vi "Mcp2210 Set Gpio Pin Val.vi"(8 "error in (no error)":errorcluster, 10 "GPIO Output":bool[](array[boolean]), 11 "handle":i32) -> (0 "error out":errorcluster, 2 "GPIO Output out":bool[](array[boolean]), 3 "handle out":i32)   [LabVIEW 2015, in "mcp2210.lvlib"]
doc: "Set the GPIO current values. Also returns back the current values.\nThe values are valid only for the pins previously configured as GPIOs.\nParameters:\nInputs:\n- void *handle - The pointer to the device handle. Cannot be NULL.\n- unsigned int gpioSetVal - GPIO pin new values.\nOutputs:\n- unsigned int *pgpioPinVal - GPIO pin values reported back, if successful call.\nIn case of error the value is not changed.\nCannot be NULL pointer.\nReturns:\n- 0 for success: E_SUCCESS\n- negative error code: E_ERR_NULL, E_ERR_INVALID_HANDLE_VALUE\nE_ERR_UNKOWN_ERROR, E_ERR_INVALID_PARAMETER\nE_ERR_HID_TIMEOUT, E_ERR_HID_RW_FILEIO\nE_ERR_CMD_ECHO, E_ERR_CMD_FAILED\n\nMCP2210_DLL_UM_API int __stdcall Mcp2210_SetGpioPinVal(void *handle, unsigned int gpioSetVal, unsigned int *pgpioPinVal);"
uses:
  <userlib>/mcp2210/mcp2210.lvlib
  <userlib>/mcp2210/mcp2210_dll_um_x86.dll
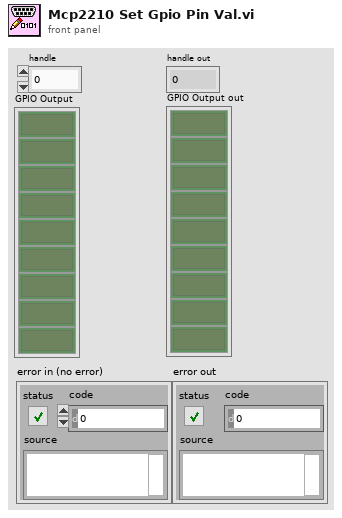
[diagram p1: front panel]
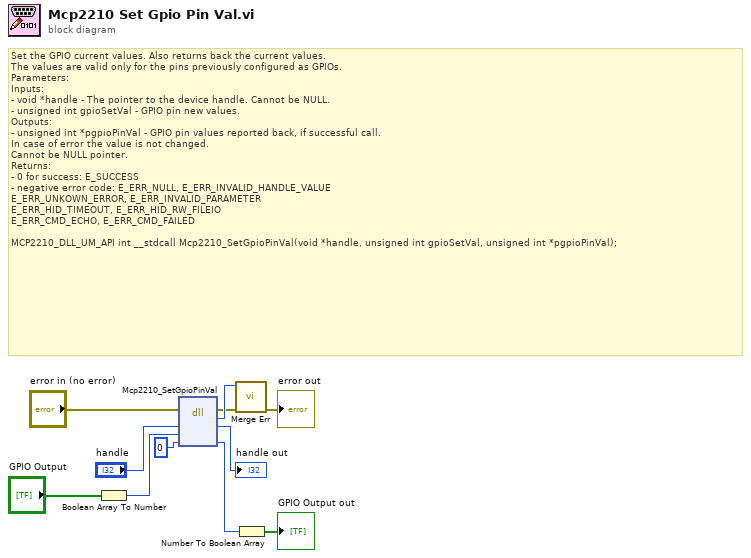
[diagram p0: block diagram]
diagram:
  # "Set the GPIO current values. Also returns back the current values.\nThe values are valid only for the pins previously configured as GPIOs.\nParameters:\nInputs:\n- void *handle - The pointer to the device handle. Cannot be NULL.\n- unsigned int gpioSetVal - GPIO pin new values.\nOutputs:\n- unsigned int *pgpioPinVal - GPIO pin values reported back, if successful call.\nIn case of error the value is not changed.\nCannot be NULL pointer.\nReturns:\n- 0 for success: E_SUCCESS\n- negative error code: E_ERR_NULL, E_ERR_INVALID_HANDLE_VALUE\nE_ERR_UNKOWN_ERROR, E_ERR_INVALID_PARAMETER\nE_ERR_HID_TIMEOUT, E_ERR_HID_RW_FILEIO\nE_ERR_CMD_ECHO, E_ERR_CMD_FAILED\n\nMCP2210_DLL_UM_API int __stdcall Mcp2210_SetGpioPinVal(void *handle, unsigned int gpioSetVal, unsigned int *pgpioPinVal);"
  n1 = Boolean Array To Number(Boolean array="GPIO Output") -> (number=w3:u32)
  n2 = dll-call lib="D:/LabVIEW 2015/user.lib/mcp2210/mcp2210_dll_um_x86.*" fn="Mcp2210_SetGpioPinVal"(error in="error in (no error)", "handle"="handle", "gpioSetVal"=w3, "pgpioPinVal"=u32 0) -> (error out=w7:errorcluster, "return type"=w8:i32, "handle"=→"handle out":i32, "pgpioPinVal"=w2:u32)  [unwired: 3 in, 1 out]
  n3 = call <userlib>:"Merge Err.vi"("error in (no error)"=w7, "return type"=w8) -> ("error out"=→"error out":errorcluster)  [unwired: 9 in]
  n4 = Number To Boolean Array(number=w2) -> (Boolean array=→"GPIO Output out":bool[])
